vi "IPI_SaveInI.vi"(7 "名称或相对路径":string="UserDefine.ini", 8 "Inputs_BaseParam":string[](array[string]), 10 "Keys":string[](array[string])=["LoadProgram"], 11 "section":string="BaseParam_Set") -> ()   [LabVIEW 2015]
uses:
  Global System.vi
  <vilib>/Utility/config.llb/NI_LVConfig.lvlib
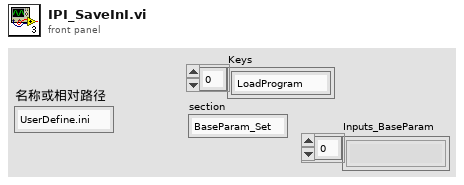
[diagram p1: front panel]
types:
  T1 = typedef "NI_LVConfig.lvlib/Config Data RefNum.ctl" = refnum<k1>
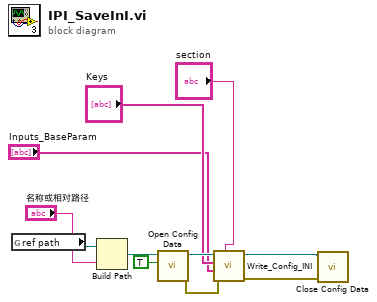
[diagram p0: block diagram]
diagram:
  n1 = global read "Global System.vi" "ref path"() -> (w6:path)
  n2 = Build Path(base path=w6, name or relative path="名称或相对路径") -> (appended path=w4:path)
  n3 = call <vilib>:"Open Config Data.vi"("create file if necessary (T)"=TRUE, "configuration file path"=w4) -> ("error out"=w10:errorcluster, "refnum"=w9:T1)  [unwired: 7 in, 1 out]
  n4 = call "Write_Config_INI.vi"("section"="section", "error in (no error)"=w10, "Inputs"="Inputs_BaseParam", "Keys"="Keys", "refnum"=w9) -> ("error out"=w1:errorcluster, "refnum 2"=w2:T1)  [unwired: 5 in]
  n5 = call <vilib>:"Close Config Data.vi"("error in (no error)"=w1, "refnum"=w2) -> ()  [unwired: 8 in, 2 out]
